vi "lv_icon.vi"(8 "error in (no error)":errorcluster, 9 "BW icon in":T1, 10 "Color icon in":T1, 11 "Class 3 in":refnum<class "Class 3.lvclass">) -> (0 "error out":errorcluster, 1 "Color icon out":T1, 2 "BW icon out":T1, 3 "Class 3 out":refnum<class "Class 3.lvclass">, 4 "Error code out":i32)   [LabVIEW 2021, in "Class 3.lvclass"]
uses:
  Class 3.lvclass
  <vilib>/picture/picture.llb/imagedata.ctl
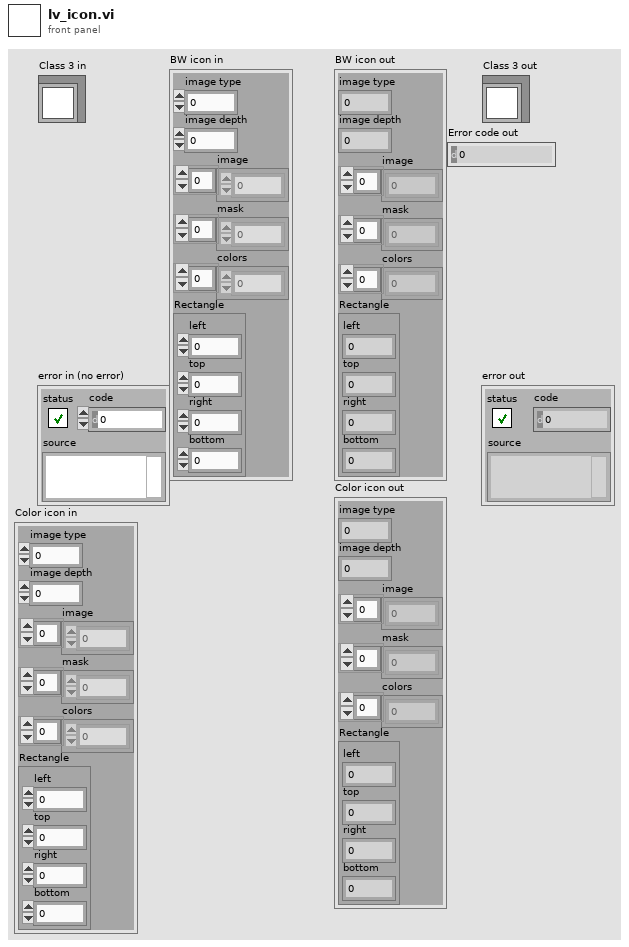
[diagram p1: front panel]
types:
  T1 = typedef "imagedata.ctl" = cluster{"image type":i32, "image depth":i32, "image":u8[], "mask":u8[], "colors":u32[], "Rectangle":cluster{"left":i16, "top":i16, "right":i16, "bottom":i16}}
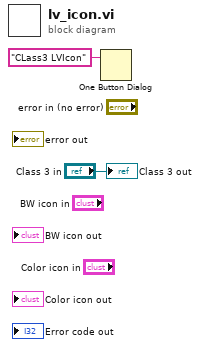
[diagram p0: block diagram]
diagram:
  n1 = One Button Dialog(message="CLass3 LVIcon") -> ()  [unwired: 1 in, 1 out]
  "Class 3 out" <- "Class 3 in"
